vi "ChessBoardIsFull.vi"(7 "ChessBoard":T1) -> (8 "Full?":bool)   [LabVIEW 2009]
uses:
  Controls/Chess.ctl
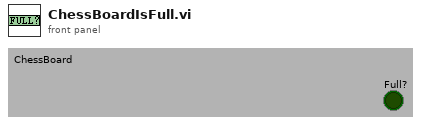
[diagram p1: front panel]
types:
  T1 = typedef "Chess.ctl" = u16[][]
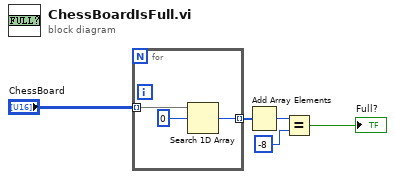
[diagram p0: block diagram]
diagram:
  n1 = for {
    tunnel: "ChessBoard" -> [w8] mode=indexing
    tunnel: [w6] -> w2 mode=indexing
    n2 = Search 1D Array(1D array=w8, element=u16 0) -> (index of element=w6:i32)  [unwired: 1 in]
  }
  n3 = Add Array Elements(numeric array=w2) -> (sum=w3:i32)
  n4 = Equal?(x=w3, y=-8) -> (x = y?=→"Full?":bool)
